vi "hReadChannels-UandP-2013.vi"(0 "FPGA VI Reference In":refnum<k20>, 1 "SavGol side points":i32=10, 3 "Use Voltage or Power for AO?":bool, 4 "order polynomial":i32=2, 5 "Nsamples":u32=10000, 6 "error in":errorcluster, 8 "output cluster":T3, 10 "variables cluster":T2) -> (2 "Fehler":bool, 13 "AdjustedArray":sgl[][](array[numeric]), 18 "single channel voltage array":dbl[](array[numeric]), 19 "real time P_rad array":dbl[](array[numeric]), 20 "FPGA VI Reference Out":refnum<k20>, 22 "PowerArray":sgl[][](array[numeric]), 25 "RawArray":sgl[][](array[numeric]), 26 "error out":errorcluster)   [LabVIEW 2014]
doc: "startet das einlesen und führt dies bis n Samples aus\nHier mit FIFO und IRQ."
uses:
  <vilib>/Utility/error.llb/Error Cluster From Error Code.vi
  <vilib>/rvi/errors/niLvFpgaAdjustHostInterfaceError.vi
  <vilib>/RVI Host/nirviSupport.llb/nirviErrorClusterFromErrorCode.vi
  <vilib>/rvi/interface/nirviReadWriteControl/nirviReadWriteControl.xnode
  FPGA Bitfiles/W7XBolo2017_FPGATarget_fmain2014_DACRangeVoltage.lvbitx
  f_main_2014.vi
  <vilib>/rvi/interface/nirviMethod/nirviMethod.xnode
  NiFpgaLv.dll
  <vilib>/rvi/interface/nirviMethod/StockFPGA_InlinedMethodWaitForMultipleIRQ.vi
  <vilib>/FPGAPlugInAG/PCI-7813R/niLvFpga_WaitOnIrq_PCI-7813R.vi
  <vilib>/FPGAPlugInAG/PCI-7813R/niLvFpga_AcknowledgeIrq_PCI-7813R.vi
  <vilib>/FPGAPlugInAG/PCI-7813R/niLvFpga_ReadFifo_PCI-7813R.vi
  <vilib>/rvi/errors/niLvFpgaMergeErrorWithErrorCode.vi
panel:
  out "channel number":i64
  in  "Tab Control":T1(tab)
  out "16bit integer voltage sample":i16[](array[numeric])
  out "RTPRad voltage factor":dbl
  out "Timed Out":bool
  out "STOP?":bool
  out "Elements Remaining":u32
  out "single channel voltage":sgl
  out "single channel voltage * factor":dbl
  out "empty sample array":dbl[](array[numeric])
  out "Nsamples array":i64[](array[numeric])
  out "dU/dt":sgl[](array[numeric])
  out "sample":i32
  out "new level of override":i32
  out "sate":string
  out "last U sample":sgl[](array[numeric])
  out "current P_rad [MW]":dbl
  out "rt prad average array":dbl[][](array[numeric])
  out "elec. channel selected":i64
  out "element of channel\nand sample":sgl
  out "column":i32
  out "channel index":i32
  out "av/f_OT*volume/k_bolo/V_cam":dbl
  out "average":dbl
  out "sum":dbl
  out "av/f_OT*volume":dbl
  out "average/f_OT":sgl
  out "av/f_OT*volume/k_bolo":dbl
  in  "magic number":dbl=1.0
  out "current power":sgl[](array[numeric])
  out "prad av array":dbl[](array[numeric])
  in  "No. Of Samples to average":i32=10
  out "index status":bool
  out "RawScal":dbl[](array[numeric])
  out "Scale(mV)":sgl[](array[numeric])
  out "SumScal":dbl[](array[numeric])
  out "Tau/dt":dbl[](array[numeric])
  out "F_ch":dbl[](array[numeric])
  out "tau_fact":dbl[](array[numeric])
  out "kbolott_and_volume":dbl[][](array[numeric])
  out "samples to exclude":u32
  out "single channel number":i64
  out "channelNumber":i32
  out "channelSelection":i64[][](array[numeric])
  out "tau_M":dbl[](array[numeric])
  out "Offsets":dbl[](array[numeric])
  out "SampleTime":sgl
  out "voltage factor":dbl
  out "Scale(mV) transf.":sgl[](array[numeric])
  out "V_cam":dbl
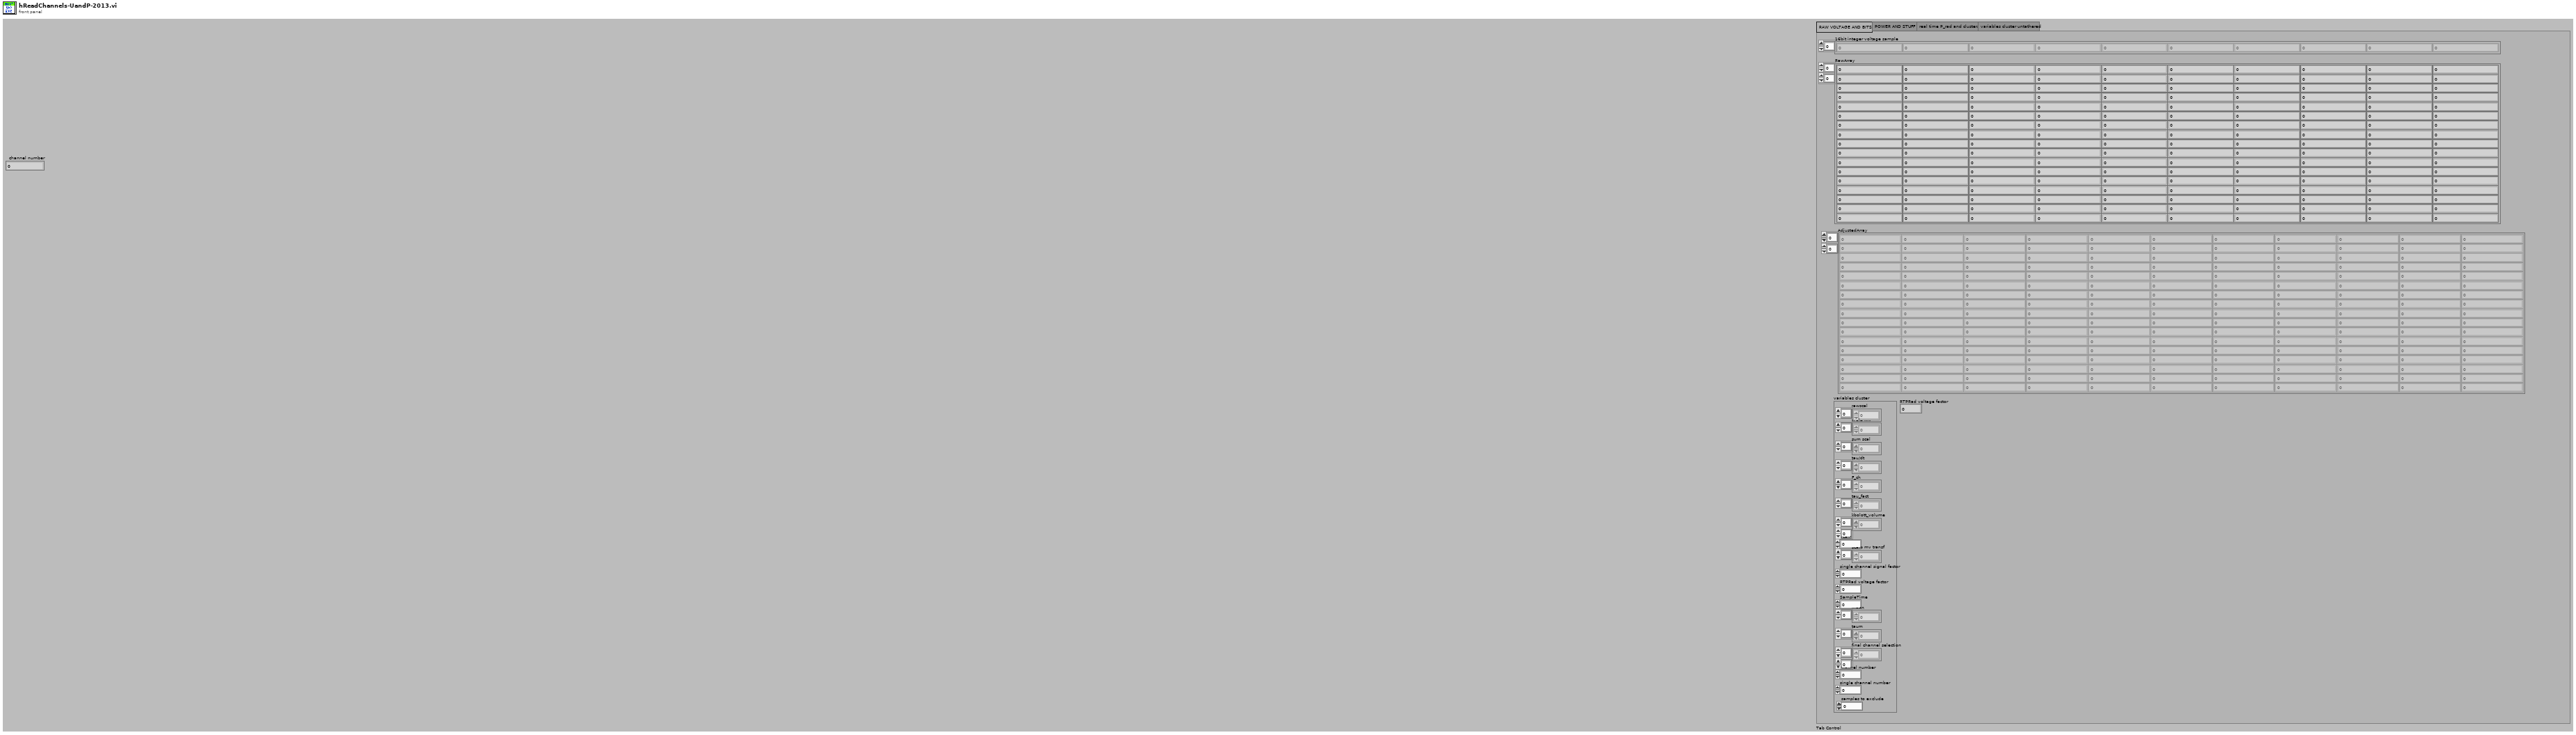
[diagram p1: front panel]
types:
  T1 = enum32{"RAW VOLTAGE AND BITS", "POWER AND STUFF", "real time P_rad and clusters", "variables cluster untathered"}
  T2 = cluster{"rawscal":dbl[], "scale mv":sgl[], "sum scal":dbl[], "tau/dt":dbl[], "F_ch":dbl[], "tau_fact":dbl[], "kbolott_volume":dbl[][], "Vcam":dbl, "scale mv transf":sgl[], "single channel signal factor":dbl, "RTPRad voltage factor":dbl, "SampleTime":sgl, "mean":dbl[], "taum":dbl[], "final channel selection":i64[][], "channel number":i32, "single channel number":i64, "samples to exclude":u32}
  T3 = cluster{"real time P_rad":refnum<vi>, "real time P_rad array":refnum<vi>, "single channel voltage":refnum<vi>, "single channel voltage array":refnum<vi>}
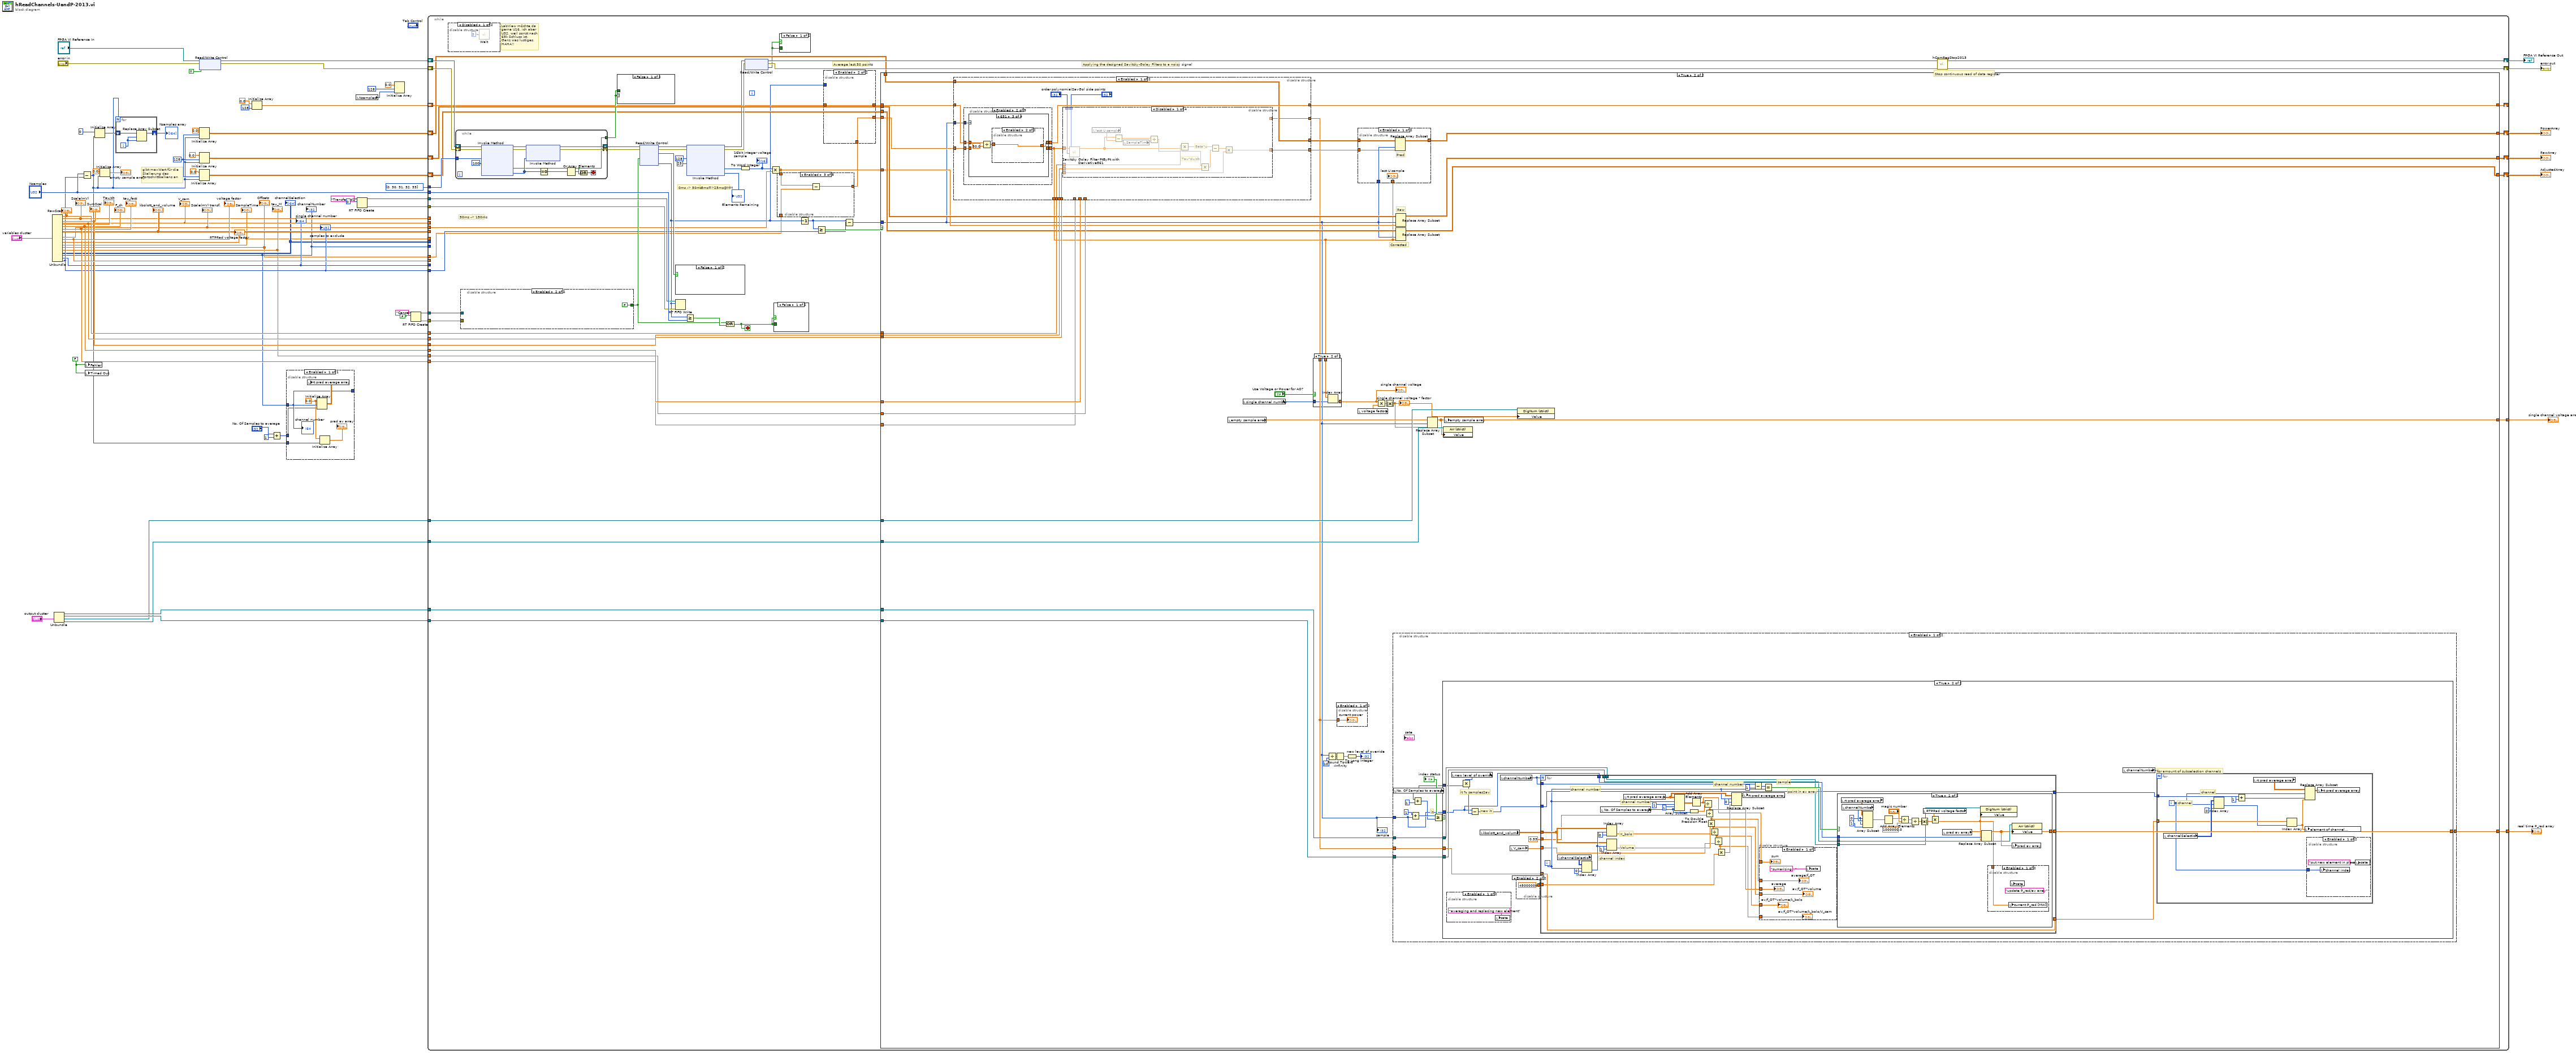
[diagram p0: block diagram]
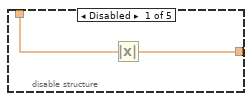
[diagram p2: hidden frame]
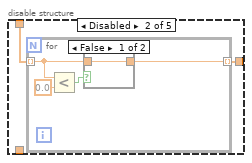
[diagram p3: hidden frame]
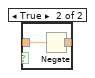
[diagram p4: hidden frame]
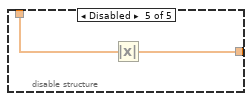
[diagram p6: hidden frame]
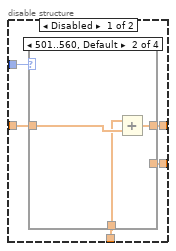
[diagram p7: hidden frame]
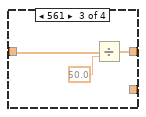
[diagram p9: hidden frame]
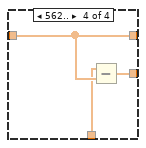
[diagram p10: hidden frame]
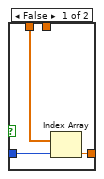
[diagram p12: hidden frame]
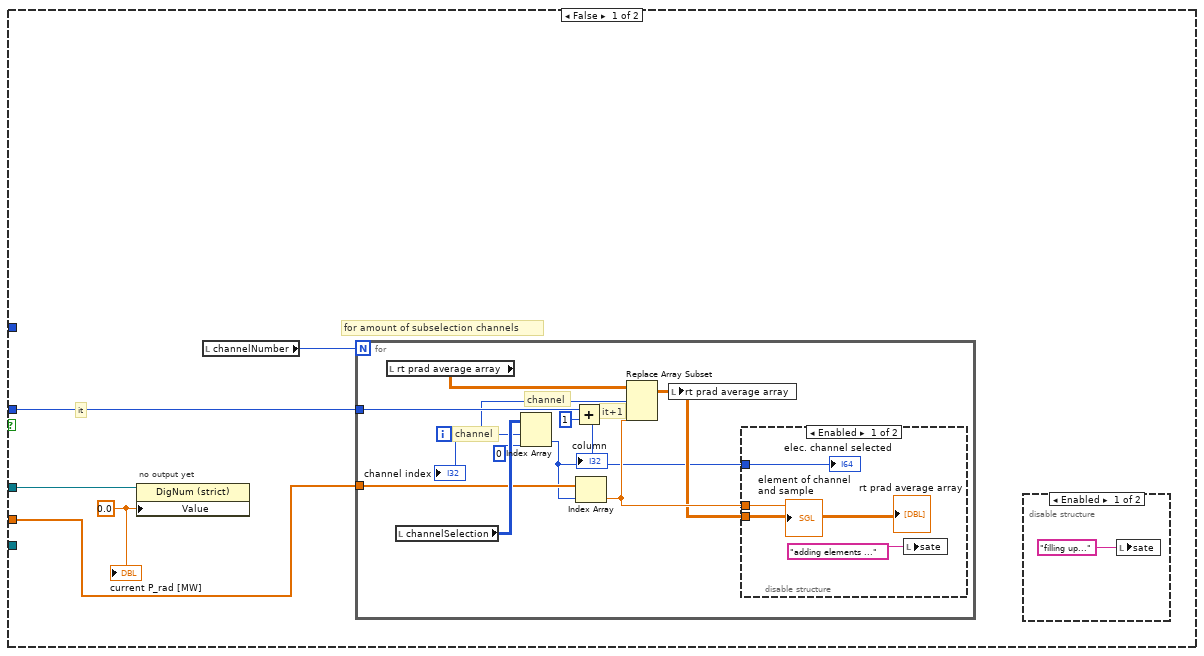
[diagram p14: hidden frame]
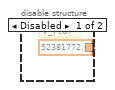
[diagram p17: hidden frame]
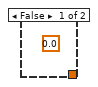
[diagram p20: hidden frame]
diagram:
  w40 = FALSE
  w14 = 128 ("dimension size")
  # "Stop continuous read of data register"
  # "gibt maxWert für die Skalierung des Fortschrittbalkens an"
  n1 = Unbundle("variables cluster") -> ("rawscal"=w31:dbl[], "scale mv"=w26:sgl[], "sum scal"=w32:dbl[], "tau/dt"=w30:dbl[], "F_ch"=w29:dbl[], "tau_fact"=w28:dbl[], "kbolott_volume"=w27:dbl[][], "Vcam"=w24:dbl, "scale mv transf"=w25:sgl[], "single channel signal factor"=w33:dbl, "RTPRad voltage factor"=→"RTPRad voltage factor":dbl, "SampleTime"=w3:sgl, "mean"=w4:dbl[], "taum"=w5:dbl[], "final channel selection"=w6:i64[][], "channel number"=w7:i32, "single channel number"=w8:i64, "samples to exclude"=w9:u32)
  "RawScal" <- w31
  "Scale(mV)" <- w26
  "SumScal" <- w32
  "Tau/dt" <- w30
  "F_ch" <- w29
  "tau_fact" <- w28
  "kbolott_and_volume" <- w27
  "V_cam" <- w24
  "Scale(mV) transf." <- w25
  "voltage factor" <- w33
  "SampleTime" <- w3
  "Offsets" <- w4
  "tau_M" <- w5
  "channelSelection" <- w6
  "channelNumber" <- w7
  "single channel number" <- w8
  "samples to exclude" <- w9
  n2 = Unbundle("output cluster") -> ("real time P_rad"=w35:refnum<vi>, "real time P_rad array"=w34:refnum<vi>, "single channel voltage"=w19:refnum<vi>, "single channel voltage array"=w18:refnum<vi>)
  n3 = Subtract(x="Nsamples", y=w9) -> (x-y=w13:u32)
  n4 = local write "Fehler"(w40) -> ()
  n5 = local write "Timed Out"(w40) -> ()
  n6 = Initialize Array(i64 0 ("element"), w13) -> (w42:i64[])
  n7 = Initialize Array(0.0 ("element"), w13) -> (→"empty sample array":dbl[])
  n8 = for {
    N: w13 -> [_]
    shift-right: [w72] -> w41
    shift-left: w42 -> [w74]
    i -> [w73]
    n9 = Replace Array Subset(array=w74, new element=w73, index=w73) -> (w72:i64[])
  }
  "Nsamples array" <- w41
  n10 = Initialize Array(sgl 0.0 ("element"), w14, w13) -> (w12:sgl[][])
  n11 = xnode "Read/Write Control"("FPGA VI Reference In"="FPGA VI Reference In", "error in"="error in", "ADCRead"=TRUE) -> ("FPGA VI Reference Out"=w53:refnum<k20>, "error out"=w52:errorcluster)
  n12 = Initialize Array(sgl 0.0 ("i"), w14, w13) -> (w62:sgl[][])
  n13 = Initialize Array(sgl 0.0, w14, w13) -> (w71:sgl[][])
  n14 = Initialize Array(sgl 0.0 ("element"), 128 ("dimension size")) -> (w48:sgl[])
  n15 = Add(x="No. Of Samples to average", y=1) -> (x+y=w21:i32)
  n16 = disable-structure shown="Enabled" {
    disable-tunnel: w7 -> [w79]
    disable-tunnel: [w79] -> _
    disable-tunnel: w21 -> [w75]
    disable-tunnel: w13 -> [w76]
    frame Enabled {
      w78 = 0.0 ("element")
      n17 = Initialize Array(w78, w79, w75) -> (w80:dbl[][])
      n18 = local write "rt prad average array"(w80) -> ()
      n19 = Initialize Array(w78, w76) -> (→"prad av array":dbl[])
      "channel number" <- w79
    }
  }
  n20 = local read "Nsamples"() -> (w37:u32)
  n21 = RT FIFO Create(0:"Transferred1" ("name (unnamed)"), 1:u32 0) -> (8:w68:refnum<k33>, 11:w67:errorcluster)  [unwired: 2 in, 5 out]
  n22 = Initialize Array(sgl 0.0 ("element"), 128 ("dimension size"), w37) -> ()  [unwired: 1 out]
  n23 = RT FIFO Create(0:"Cancel" ("name (unnamed)"), 1:FALSE) -> (8:w65:refnum<k33>, 11:w64:errorcluster)  [unwired: 2 in, 5 out]
  n24 = while {
    tunnel: "Nsamples" -> [w133]
    shift-right: [w101] -> w10
    shift-left: w71 -> [w122]
    shift-right: [w134] -> w61
    shift-left: w53 -> [w137]
    shift-right: [w135] -> w60
    shift-left: w52 -> [w136]
    tunnel: w68 -> [w132]
    tunnel: w67 -> [w131]
    tunnel: w65 -> [w129]
    tunnel: w64 -> [w128]
    shift-right: [w126] -> w56
    shift-left: w62 -> [w127]
    tunnel: w25 -> [w121]
    tunnel: w30 -> [w118]
    tunnel: w32 -> [w120]
    tunnel: w31 -> [w119]
    shift-right: [w111] -> _
    shift-left: w48 -> [w87]
    tunnel: i32[] [0, 30, 31, 32, 33] -> [w106]
    tunnel: w18 -> [w103]
    tunnel: w19 -> [w102]
    tunnel: w8 -> [_]
    tunnel: w33 -> [_]
    tunnel: w4 -> [w81]
    tunnel: w9 -> [w82]
    tunnel: w35 -> [w98]
    tunnel: w34 -> [w93]
    tunnel: w29 -> [w97]
    tunnel: w28 -> [w96]
    tunnel: w26 -> [_]
    tunnel: w27 -> [_]
    tunnel: w3 -> [_]
    tunnel: w5 -> [w95]
    tunnel: w6 -> [_]
    tunnel: w7 -> [_]
    tunnel: w24 -> [_]
    tunnel: [w92] -> w17
    tunnel: [w91] -> w16
    shift-right: [w89] -> w11
    shift-left: w12 -> [w90]
    stop <- w107 stop-if-true
    # "Average last 50 points"
    # "Applying the designed Savitzky-Golay Filters to a noisy signal"
    # "LabView möchte da gerne U16, ich aber U32, weil sonst nach 65k Schluss ist. \nGanz was lustiges, HAHA!!"
    # "5ms=>25ms@MM"
    # "0ms -> 50ms"
    # "50ms -> 150ms"
    n25 = disable-structure shown="Disabled" {
      frame Disabled {
        n26 = call "Wait"("Count(uSec)"=u32 5) -> ()  [unwired: 1 out]
      }
      frame Enabled {
      }
    }
    n27 = while {
      tunnel: [w513] -> w110
      shift-right: [w515] -> w104
      shift-left: w137 -> [w522]
      shift-right: [w514] -> w105
      shift-left: w136 -> [w521]
      tunnel: w106 -> [w519]
      stop <- w512 stop-if-true
      n28 = xnode "Invoke Method"("FPGA VI Reference In"=w522, "error in"=w521, "IRQ Number(s)"=w519, "Timeout (ms)"=100) -> ("FPGA VI Reference Out"=w516:refnum<k20>, "error out"=w517:errorcluster, "Timed Out"=w513:bool, "IRQ(s) Asserted"=w518:i32[])
      n29 = xnode "Invoke Method"("FPGA VI Reference In"=w516, "error in"=w517, "IRQ Number(s)"=w518) -> ("FPGA VI Reference Out"=w515:refnum<k20>, "error out"=w514:errorcluster)
      n30 = Equal To 0?(x=w518) -> (x = 0?=w511:bool[])
      n31 = Or Array Elements(Boolean array=w511) -> (logical OR=w510:bool)
      n32 = Or(x=w510, y=w513) -> (x .or. y?=w512:bool)
    }
    n33 = disable-structure shown="Enabled" {
      disable-tunnel: [w528 FALSE] -> w130
      disable-tunnel: w129 -> [w527 _]
      disable-tunnel: w128 -> [w526 _]
      frame Disabled {
        # "Da es passieren kann, dass der letzte IRQ verschluckt wird, sichert dies der Timeoutwert von 50ms ab."
        n34 = RT FIFO Read(0:w527, 1:FALSE ("element"), 3:w526) -> (9:w528:bool)  [unwired: 5 out]
      }
      frame Enabled {
      }
    }
    n35 = case shown="False" w110 {
      tunnel: w110 -> [_ w530]
      frame False {
      }
      frame True {
        "Timed Out" <- w530
      }
    }
    n36 = xnode "Read/Write Control"("FPGA VI Reference In"=w104, "error in"=w105, "cancel"=w130) -> ("FPGA VI Reference Out"=w124:refnum<k20>, "error out"=w123:errorcluster, "Timeout"=w125:bool, "ScanID"=w88:u32)
    n37 = case shown="False" w125 {
      selector: w125 -> [_ w532]
      frame False {
      }
      frame True {
        n38 = local write "Fehler"(w532) -> ()
      }
    }
    n39 = RT FIFO Write(0:w132, 1:w88, 3:w131) -> ()  [unwired: 1 in, 5 out]
    n40 = Greater Or Equal?(x=w88, y=w133) -> (x >= y?=w138:bool)
    n41 = xnode ("Invoke Method")("FPGA VI Reference In"=w124, "error in"=w123, "Number of Elements"=u32 128, "Timeout (ms)"=25 ("Timeout")) -> ("FPGA VI Reference Out"=w113:refnum<k20>, "error out"=w112:errorcluster, "Data"=w115:u32[], "Elements Remaining"=→"Elements Remaining":u32)
    n42 = Compound Arithmetic op=OR(w130, w138) -> (w107:bool)
    n43 = To Word Integer(number=w115) -> (16bit integer=w114:i16[])
    "16bit integer voltage sample" <- w114
    n44 = xnode "Read/Write Control"("FPGA VI Reference In"=w113, "error in"=w112) -> ("FPGA VI Reference Out"=w134:refnum<k20>, "error out"=w135:errorcluster, "Fifo-Fehler"=w108:bool)
    n45 = Multiply(x=w114, y=w121) -> (x*y=w85:sgl[])
    n46 = case shown="False" w107 {
      tunnel: w107 -> [_ w523]
      frame False {
      }
      frame True {
        "STOP?" <- w523
      }
    }
    n47 = disable-structure shown="Enabled" {
      disable-tunnel: [w140 w141 w152 w153 w155] -> w84
      disable-tunnel: w85 -> [w139 w142 w151 w153 w154]
      disable-tunnel: w81 -> [_ _ w150 _ _]
      frame Disabled {
        n48 = Absolute Value(x=w139) -> (abs(x)=w140:sgl[])
      }
      frame Disabled {
        n49 = for {
          tunnel: w142 -> [w144] mode=indexing
          tunnel: [w143] -> w141 mode=indexing
          n50 = Less?(x=w144, y=sgl 0.0) -> (x < y?=w145:bool)
          n51 = case shown="False" w145 {
            tunnel: w144 -> [w147 w149]
            tunnel: [w147 w148] -> w143
            frame False {
            }
            frame True {
              n52 = Negate(x=w149) -> (-x=w148:sgl)
            }
          }
        }
      }
      frame Enabled {
        n53 = Subtract(x=w151, y=w150) -> (x-y=w152:dbl[])
      }
      frame Disabled {
      }
      frame Disabled {
        n54 = Absolute Value(x=w154) -> (abs(x)=w155:sgl[])
      }
    }
    n55 = case shown="False" w108 {
      tunnel: w108 -> [_ w524]
      frame False {
      }
      frame True {
        "Fehler" <- w524
      }
    }
    n56 = Decrement(x=w88) -> (x-1=w99:u32)
    n57 = Greater Or Equal?(x=w99, y=w82) -> (x >= y?=w100:bool)
    n58 = disable-structure shown="Enabled" {
      disable-tunnel: [w160 w172] -> w86
      disable-tunnel: w87 -> [w159 w172]
      disable-tunnel: w88 -> [w158 _]
      disable-tunnel: [w157 w171] -> w83
      disable-tunnel: w84 -> [w156 w171]
      frame Disabled {
        n59 = case shown="501..560, Default" w158 {
          tunnel: w156 -> [_ w162 _ w168]
          tunnel: [w161 w164 w165 w169] -> w160
          tunnel: w159 -> [w161 w163 w167 w169]
          tunnel: [_ _ _ w170] -> w157
          frame 0..500 {
          }
          frame 501..560, Default {
            n60 = Add(x=w162, y=w163) -> (x+y=w164:dbl[])
          }
          frame 561 {
            n61 = Divide(x=w167, y=sgl 50.0) -> (x/y=w165:dbl[])
          }
          frame 562.. {
            n62 = Subtract(x=w168, y=w169) -> (x-y=w170:dbl[])
          }
        }
      }
      frame Enabled {
      }
    }
    n63 = Subtract(x=w99, y=w82) -> (x-y=w94:u32)
    n64 = case shown="True" w100 {
      tunnel: w127 -> [w175 w214]
      tunnel: [w175 w207] -> w126
      tunnel: w122 -> [w174 w205]
      tunnel: w120 -> [_ w213]
      tunnel: w119 -> [_ w212]
      tunnel: w118 -> [_ w211]
      tunnel: [w176 w210] -> w111
      tunnel: w86 -> [w176 w184]
      tunnel: w85 -> [_ w183]
      tunnel: w103 -> [_ w209]
      tunnel: w102 -> [_ w208]
      tunnel: [w174 w204] -> w101
      tunnel: w94 -> [_ w181]
      tunnel: w98 -> [_ w200]
      tunnel: w93 -> [_ w199]
      tunnel: w97 -> [_ w203]
      tunnel: w96 -> [_ w201]
      tunnel: w95 -> [_ w202]
      tunnel: [_ w189] -> w92
      tunnel: [_ w188] -> w91
      tunnel: w90 -> [w173 w186]
      tunnel: [w173 w185] -> w89
      tunnel: w83 -> [_ w182]
      frame False {
      }
      frame True {
        # "Corrected"
        # "Raw"
        n65 = disable-structure shown="Enabled" {
          disable-tunnel: w214 -> [w362 w477]
          disable-tunnel: w213 -> [w369 _]
          disable-tunnel: w212 -> [w368 _]
          disable-tunnel: w211 -> [w367 _]
          disable-tunnel: [w366 w473] -> w210
          disable-tunnel: w184 -> [w365 w475]
          disable-tunnel: w182 -> [w359 w474]
          disable-tunnel: w181 -> [w364 w476]
          disable-tunnel: w202 -> [_ w483]
          disable-tunnel: w203 -> [_ w482]
          disable-tunnel: w201 -> [_ w481]
          disable-tunnel: [w363 w479] -> w178
          disable-tunnel: [w362 w477] -> w206
          disable-tunnel: [w358 _] -> w179
          disable-tunnel: [w357 _] -> w177
          frame Enabled {
            n66 = disable-structure shown="Enabled" {
              disable-tunnel: [w374 w400 w422] -> w366
              disable-tunnel: w365 -> [w373 w399 w422]
              disable-tunnel: w364 -> [w372 w398 _]
              disable-tunnel: [w371 w397 w423] -> w358
              disable-tunnel: w359 -> [w370 w396 w423]
              frame Disabled {
                n67 = case shown="11..60, Default" w372 {
                  tunnel: w370 -> [_ w376 _ w392]
                  tunnel: [w375 w378 w380 w391] -> w374
                  tunnel: w373 -> [w375 w377 w382 w391]
                  tunnel: [_ _ _ w390] -> w371
                  frame 0..10 {
                  }
                  frame 11..60, Default {
                    # "Average last 50 points"
                    n68 = Add(x=w376, y=w377) -> (x+y=w378:dbl[])
                  }
                  frame 61 {
                    n69 = Divide(x=w382, y=sgl 50.0) -> (x/y=w379:dbl[])
                    n70 = disable-structure shown="Enabled" {
                      disable-tunnel: [w383 w388] -> w380
                      disable-tunnel: w379 -> [w387 w388]
                      frame Disabled {
                        n71 = Initialize Array(2e-06 ("element"), 128 ("dimension size")) -> (w384:dbl[])
                        n72 = Subtract(x=w387, y=w384) -> (x-y=w383:dbl[])
                      }
                      frame Enabled {
                      }
                    }
                  }
                  frame 62.. {
                    n73 = Subtract(x=w392, y=w391) -> (x-y=w389:dbl[])
                    n74 = disable-structure shown="Enabled" {
                      disable-tunnel: [w394 w395] -> w390
                      disable-tunnel: w389 -> [w393 w395]
                      frame Disabled {
                        n75 = Absolute Value(x=w393) -> (abs(x)=w394:dbl[])
                      }
                      frame Enabled {
                      }
                    }
                  }
                }
              }
              frame Enabled {
                n76 = case shown="651" w398 {
                  tunnel: w396 -> [_ w402 _ w418]
                  tunnel: [w401 w404 w406 w417] -> w400
                  tunnel: w399 -> [w401 w403 w408 w417]
                  tunnel: [_ _ _ w416] -> w397
                  frame 0..600 {
                  }
                  frame 601..650, Default {
                    # "Average last 50 points"
                    n77 = Add(x=w402, y=w403) -> (x+y=w404:dbl[])
                  }
                  frame 651 {
                    n78 = Divide(x=w408, y=sgl 50.0) -> (x/y=w405:dbl[])
                    n79 = disable-structure shown="Enabled" {
                      disable-tunnel: [w409 w414] -> w406
                      disable-tunnel: w405 -> [w413 w414]
                      frame Disabled {
                        n80 = Initialize Array(2e-06 ("element"), 128 ("dimension size")) -> (w410:dbl[])
                        n81 = Subtract(x=w413, y=w410) -> (x-y=w409:dbl[])
                      }
                      frame Enabled {
                      }
                    }
                  }
                  frame 652.. {
                    n82 = Subtract(x=w418, y=w417) -> (x-y=w415:dbl[])
                    n83 = disable-structure shown="Enabled" {
                      disable-tunnel: [w420 w421] -> w416
                      disable-tunnel: w415 -> [w419 w421]
                      frame Disabled {
                        n84 = Absolute Value(x=w419) -> (abs(x)=w420:dbl[])
                      }
                      frame Enabled {
                      }
                    }
                  }
                }
              }
              frame Disabled {
              }
            }
            n85 = disable-structure shown="Disabled" {
              disable-tunnel: w369 -> [w438 w450 w456 _]
              disable-tunnel: w368 -> [w437 w449 w451 _]
              disable-tunnel: w367 -> [w436 w448 w455 _]
              disable-tunnel: [w435 w439 w470 w471] -> w363
              disable-tunnel: w358 -> [w434 w447 w469 w471]
              disable-tunnel: "SavGol side points" -> [w428 w442 w463 _]
              disable-tunnel: "order polynomial" -> [w429 w443 w464 _]
              disable-tunnel: [_ w439 w453 w471] -> w357
              frame Disabled {
                # "Beta*u"
                # "Tau*du/dt"
                n86 = call "Savitzky Golay Filter PtByPt with Derivative861.vi"("order polynomial"=w429, "side points"=w428, "x"=w434) -> ("Filtered x"=w424:dbl[])  [unwired: 1 in, 7 out]
                n87 = local read "last U sample"() -> (w426:sgl[])
                n88 = Subtract(x=w424, y=w426) -> (x-y=w427:dbl[])
                n89 = local read "SampleTime"() -> (w425:sgl)
                n90 = Divide(x=w427, y=w425) -> (x/y=w431:dbl[])
                n91 = Multiply(x=w437, y=w424) -> (x*y=w433:dbl[])
                n92 = Multiply(x=w431, y=w436) -> (x*y=w430:dbl[])
                n93 = Subtract(x=w433, y=w430) -> (x-y=w432:dbl[])
                n94 = Multiply(x=w432, y=w438) -> (x*y=w435:dbl[])
              }
              frame Enabled {
                # "Beta*u"
                # "Tau*du/dt"
                n95 = call "Savitzky Golay Filter PtByPt with Derivative861.vi"("order polynomial"=w443, "side points"=w442, "x"=w447) -> ("Filtered Derivative"=w440:dbl[], "Filtered x"=w441:dbl[])  [unwired: 1 in, 6 out]
                n96 = Multiply(x=w449, y=w441) -> (x*y=w446:dbl[])
                n97 = Multiply(x=w440, y=w448) -> (x*y=w444:dbl[])
                n98 = Subtract(x=w446, y=w444) -> (x-y=w445:dbl[])
                n99 = Multiply(x=w445, y=w450) -> (x*y=w439:dbl[])
              }
              frame Disabled {
                # "Beta*u"
                # "Tau*du/dt"
                n100 = call "Savitzky Golay Filter PtByPt with Derivative861.vi"("order polynomial"=w464, "side points"=w463, "x"=w469) -> ("Filtered Derivative"=w454:dbl[], "Filtered x"=w452:dbl[])  [unwired: 1 in, 6 out]
                n101 = local read "last U sample"() -> (w461:sgl[])
                n102 = Subtract(x=w452, y=w461) -> (x-y=w462:dbl[])
                n103 = local read "SampleTime"() -> (w460:sgl)
                n104 = Divide(x=w462, y=w460) -> (x/y=w466:dbl[])
                n105 = Multiply(x=w451, y=w452) -> (x*y=w459:dbl[])
                n106 = Multiply(x=w451, y=w452) -> (x*y=w468:dbl[])
                n107 = Multiply(x=w454, y=w455) -> (x*y=w457:dbl[])
                n108 = Multiply(x=w466, y=w455) -> (x*y=w465:dbl[])
                n109 = Subtract(x=w459, y=w457) -> (x-y=w458:dbl[])
                n110 = Subtract(x=w468, y=w465) -> (x-y=w467:dbl[])
                n111 = Multiply(x=w458, y=w456) -> (x*y=w453:dbl[])
                n112 = Multiply(x=w467, y=w456) -> (x*y=w470:dbl[])
              }
              frame Disabled {
              }
            }
          }
          frame Disabled {
            # "beta=[1-(omega*R_ch)^2+(omega*r_C)^2]/\n         {1+[omega*{R_ch+r_C}]^2}"
            # "tau_fact[((1-U_eff^2*beta)/4)/kappa_ch]/{R_ch+r_C}^2"
            # "U_eff=(U_0*R_Ch)/(R_ch+2*r_C)"
            # "omega=2*Pi*f_bridge*C_Cab"
            # "=2/U_eff * (R_ch+r_C)*kappa_ch\n  * sqrt(1+[omega+(R_ch+r_C)]^2)\n  * {tau_ch*dU/dt+tau_fact*U_ch}"
            # "P_ch=F_Ch*(tau_ch*dU/dt+tau_fact*U_ch)"
            # "tau_channels"
            # "F_ch"
            # "tau_fact"
            # "U_raw"
            # "dU/dt"
            n113 = case shown="62.." w476 {
              tunnel: w474 -> [_ w491 _ w497]
              tunnel: [w489 w492 w494 w498] -> w473
              tunnel: w475 -> [w489 w490 w495 w498]
              tunnel: [w489 _ _ w496] -> w472
              frame 0..10 {
              }
              frame 11..60, Default {
                # "Average last 50 points"
                n114 = Add(x=w491, y=w490) -> (x+y=w492:dbl[])
              }
              frame 61 {
                n115 = Divide(x=w495, y=sgl 50.0) -> (x/y=w494:dbl[])
              }
              frame 62.. {
                n116 = Subtract(x=w497, y=w498) -> (x-y=w496:dbl[])
              }
            }
            n117 = local read "last U sample"() -> (w478:sgl[])
            n118 = local read "SampleTime"() -> (w480:sgl)
            n119 = disable-structure shown="Enabled" {
              disable-tunnel: w472 -> [w504 w505]
              disable-tunnel: [w503 w506] -> w485
              disable-tunnel: [w500 w505] -> w484
              disable-tunnel: w478 -> [_ w509]
              disable-tunnel: w480 -> [_ w507]
              frame Enabled {
                n120 = call "Savitzky Golay Filter PtByPt with Derivative861.vi"("order polynomial"=2, "side points"=11, "x"=w504) -> ("Filtered Derivative"=w503:dbl[], "Filtered x"=w500:dbl[])  [unwired: 1 in, 6 out]
              }
              frame Disabled {
                # "differentiation"
                n121 = Subtract(x=w505, y=w509) -> (x-y=w508:dbl[])
                n122 = Divide(x=w508, y=w507) -> (x/y=w506:dbl[])
              }
            }
            n123 = disable-structure shown="Enabled" {
              disable-tunnel: w485 -> [w499 _]
              frame Enabled {
                "dU/dt" <- w499
              }
              frame Disabled {
              }
            }
            n124 = Multiply(x=w484, y=w481) -> (x*y=w488:dbl[])
            n125 = Multiply(x=w485, y=w483) -> (x*y=w486:dbl[])
            n126 = Add(x=w488, y=w486) -> (x+y=w487:dbl[])
            n127 = Multiply(x=w487, y=w482) -> (x*y=w479:dbl[])
          }
        }
        n128 = local read "empty sample array"() -> (w196:dbl[])
        n129 = local read "single channel number"() -> (w198:i64)
        n130 = case shown="True" "Use Voltage or Power for AO?" {
          tunnel: w198 -> [w215 w220]
          tunnel: [w216 w219] -> w195
          tunnel: w179 -> [_ w218]
          tunnel: w177 -> [w217 _]
          frame False {
            n131 = Index Array(array=w217, index=w215) -> (element=w216:dbl)
          }
          frame True {
            n132 = Index Array(array=w218, index=w220) -> (element=w219:dbl)
          }
        }
        "single channel voltage" <- w195
        n133 = Divide(x=w181, y=10) -> (x/y=w191:dbl)
        n134 = Round Toward -Infinity(1:w191) -> (0:w192:dbl)
        n135 = disable-structure shown="Enabled" {
          disable-tunnel: w177 -> [w221 _]
          frame Enabled {
            "current power" <- w221
          }
          frame Disabled {
          }
        }
        n136 = To Long Integer(number=w192) -> (32bit integer=→"new level of override":i32)
        n137 = disable-structure shown="Enabled" {
          disable-tunnel: w206 -> [w355 w356]
          disable-tunnel: [w354 w356] -> w207
          disable-tunnel: w181 -> [w353 _]
          disable-tunnel: w178 -> [w352 _]
          disable-tunnel: w179 -> [w351 _]
          frame Enabled {
            # "Prad"
            n138 = Replace Array Subset(array=w355, new element=w352, index (col)=w353) -> (w354:sgl[][])  [unwired: 1 in]
            "last U sample" <- w351
          }
          frame Disabled {
          }
        }
        n139 = local read "voltage factor"() -> (w197:dbl)
        n140 = Multiply(x=w195, y=w197) -> (x*y=w194:dbl)
        n141 = Absolute Value(x=w194) -> (abs(x)=w180:dbl)
        "single channel voltage * factor" <- w180
        n142 = disable-structure shown="Enabled" {
          disable-tunnel: w181 -> [w226 _]
          disable-tunnel: w200 -> [w229 _]
          disable-tunnel: w199 -> [w228 _]
          disable-tunnel: w177 -> [w227 _]
          disable-tunnel: [w222 _] -> w189
          frame Enabled {
            # "it"
            n143 = local read "No. Of Samples to average"() -> (w223:i32)
            n144 = Add(x=1, y=w226) -> (x+y=w230:u32)
            n145 = Add(x=w223, y=i64 1) -> (x+y=w224:i64)
            n146 = Greater Or Equal?(x=w230, y=w224) -> (x >= y?=w232:bool)
            "index status" <- w232
            n147 = case shown="True" w232 {
              tunnel: w226 -> [w233 w256]
              tunnel: w229 -> [w236 w258]
              tunnel: w228 -> [_ w259]
              tunnel: w227 -> [w234 w257]
              tunnel: w223 -> [_ w255]
              tunnel: [_ w254] -> w222
              frame False {
                w235 = 0.0 ("Value")
                # "it"
                # "for amount of subselection channels"
                # "no output yet"
                n148 = property class="DigNum (strict)"(reference=w236, "Value"=w235) -> ()  [unwired: 1 in, 2 out]
                n149 = local read "channelNumber"() -> (w237:i32)
                n150 = for {
                  N: w237 -> [_]
                  tunnel: w233 -> [w245]
                  tunnel: w234 -> [w243]
                  i -> [w240]
                  # "channel"
                  # "channel"
                  # "it+1"
                  n151 = local read "rt prad average array"() -> (w244:dbl[][])
                  n152 = local read "channelSelection"() -> (w249:i64[][])
                  n153 = Index Array(array=w249, index (row)=w240, index (col)=0 ("disabled index (col)")) -> (element=w239:i64)
                  n154 = Add(x=w245, y=1) -> (x+y=w246:u32)
                  "column" <- w246
                  n155 = Index Array(array=w243, index=w239) -> (element=w242:dbl)
                  n156 = Replace Array Subset(array=w244, new element=w242, index (row)=w240, index (col)=w246) -> (w241:dbl[][])
                  n157 = local write "rt prad average array"(w241) -> ()
                  n158 = disable-structure shown="Enabled" {
                    disable-tunnel: w239 -> [w252 _]
                    disable-tunnel: w242 -> [w251 _]
                    disable-tunnel: w241 -> [w250 _]
                    frame Enabled {
                      n159 = local write "sate"("adding elements ...") -> ()
                      "element of channel\nand sample" <- w251
                      "elec. channel selected" <- w252
                      "rt prad average array" <- w250
                    }
                    frame Disabled {
                    }
                  }
                  "channel index" <- w240
                }
                n160 = disable-structure shown="Enabled" {
                  frame Enabled {
                    n161 = local write "sate"("filling up...") -> ()
                  }
                  frame Disabled {
                  }
                }
                "current P_rad [MW]" <- w235
              }
              frame True {
                # "new it"
                # "it % samples2av"
                # "for amount of subselection channels"
                n162 = disable-structure shown="Enabled" {
                  frame Enabled {
                    n163 = local write "sate"("averaging and replacing new element") -> ()
                  }
                  frame Disabled {
                  }
                }
                n164 = local read "new level of override"() -> (w269:i32)
                n165 = Multiply(x=w269, y=w255) -> (x*y=w268:i32)
                n166 = Subtract(x=w256, y=w268) -> (x-y=w266:u32)
                n167 = local read "kbolott_and_volume"() -> (w267:dbl[][])
                n168 = local read "channelNumber"() -> (w261:i32)
                n169 = local read "V_cam"() -> (w263:dbl)
                n170 = disable-structure shown="Enabled" {
                  disable-tunnel: [52381772.0 45000000.0] -> w265
                  frame Disabled {
                    # "V_Ptor"
                  }
                  frame Enabled {
                  }
                }
                n171 = for {
                  N: w261 -> [_]
                  tunnel: w267 -> [w305]
                  tunnel: [w310] -> w262
                  tunnel: w257 -> [w310]
                  tunnel: [w290] -> w260
                  tunnel: w266 -> [w290]
                  tunnel: w265 -> [w284]
                  tunnel: 0.53 -> [w288]
                  tunnel: w263 -> [w285]
                  tunnel: w261 -> [w291]
                  tunnel: w256 -> [w296]
                  tunnel: w259 -> [w295]
                  tunnel: w258 -> [w292]
                  tunnel: [w274] -> w254
                  i -> [w289]
                  # "channel number"
                  # "channel number"
                  # "point in av array"
                  # "sample"
                  # "channel number"
                  # "K_bolo"
                  # "Volume"
                  # "channel index"
                  n172 = local read "channelSelection"() -> (w309:i64[][])
                  n173 = Index Array(array=w309, index (row)=w289, index (col)=0 ("disabled index (col)")) -> (element=w306:i64)
                  n174 = local read "No. Of Samples to average"() -> (w276:i32)
                  n175 = Index Array(array=w305, index (row)=w306, index (col)=0 ("disabled index (col)")) -> (element=w286:dbl)
                  n176 = Index Array(array=w305, index (row)=w306, index (col)=1 ("disabled index (col)")) -> (element=w287:dbl)
                  n177 = local read "rt prad average array"() -> (w300:dbl[][])
                  n178 = Array Subset(array=w300, index (row)=w289, length (row)=1, index (col)=1 ("index"), length (col)=w276) -> (w301:dbl[][])
                  n179 = To Double Precision Float(number=w276) -> (double precision float=w275:dbl)
                  n180 = Add Array Elements(numeric array=w301) -> (sum=w281:dbl)
                  n181 = Divide(x=w281, y=w275) -> (x/y=w282:dbl)
                  n182 = Divide(x=w282, y=w288) -> (x/y=w280:dbl)
                  n183 = Multiply(x=w280, y=w287) -> (x*y=w279:dbl)
                  n184 = Divide(x=w279, y=w286) -> (x/y=w278:dbl)
                  n185 = Divide(x=w278, y=w285) -> (x/y=w277:dbl)
                  n186 = Multiply(x=w277, y=w284) -> (x*y=w283:dbl)
                  n187 = Replace Array Subset(array=w300, new element=w283, index (row)=w289, index (col)=0 ("disabled index (col)")) -> (w298:dbl[][])
                  n188 = local write "rt prad average array"(w298) -> ()
                  n189 = Subtract(x=w291, y=i64 1) -> (x-y=w294:i64)
                  n190 = disable-structure shown="Enabled" {
                    disable-tunnel: w282 -> [w316 _]
                    disable-tunnel: w281 -> [w315 _]
                    disable-tunnel: w280 -> [w314 _]
                    disable-tunnel: w279 -> [w313 _]
                    disable-tunnel: w278 -> [w312 _]
                    disable-tunnel: w277 -> [w311 _]
                    frame Enabled {
                      n191 = local write "sate"("sumarizing...") -> ()
                      "av/f_OT*volume/k_bolo" <- w312
                      "average/f_OT" <- w314
                      "av/f_OT*volume" <- w313
                      "sum" <- w315
                      "average" <- w316
                      "av/f_OT*volume/k_bolo/V_cam" <- w311
                    }
                    frame Disabled {
                    }
                  }
                  n192 = Equal?(x=w294, y=w289) -> (x = y?=w297:bool)
                  n193 = case shown="True" w297 {
                    tunnel: w296 -> [_ w332]
                    tunnel: w295 -> [_ w331]
                    tunnel: w292 -> [_ w330]
                    tunnel: [_ w321] -> w274
                    frame False {
                      (unwired) 0.0
                    }
                    frame True {
                      w327 = 0 ("index")
                      n194 = local read "rt prad average array"() -> (w333:dbl[][])
                      n195 = local read "channelNumber"() -> (w328:i32)
                      n196 = Array Subset(array=w333, index (row)=w327, length (row)=w328, index (col)=w327, length (col)=1 ("index")) -> (w335:dbl[][])
                      n197 = Add Array Elements(numeric array=w335) -> (sum=w325:dbl)
                      n198 = Divide(x=w325, y="magic number") -> (x/y=w326:dbl)
                      n199 = Divide(x=w326, y=1000000.0) -> (x/y=w322:dbl)
                      n200 = Absolute Value(x=w322) -> (abs(x)=w320:dbl)
                      n201 = local read "RTPRad voltage factor"() -> (w318:dbl)
                      n202 = Multiply(x=w318, y=w320) -> (x*y=w319:dbl)
                      n203 = local read "prad av array"() -> (w323:dbl[])
                      n204 = property class="DigNum (strict)"(reference=w330, "Value"=w319) -> ()  [unwired: 1 in, 2 out]
                      n205 = Replace Array Subset(array=w323, new element=w319, index=w332) -> (w321:dbl[])
                      n206 = disable-structure shown="Enabled" {
                        disable-tunnel: w319 -> [w336 _]
                        frame Enabled {
                          n207 = local write "current P_rad [MW]"(w336) -> ()
                          n208 = local write "sate"("update P_rad/av array") -> ()
                        }
                        frame Disabled {
                        }
                      }
                      n209 = property class="Arr (strict)"(reference=w331, "Value"=w321) -> ()  [unwired: 1 in, 2 out]
                      n210 = local write "prad av array"(w321) -> ()
                    }
                  }
                }
                n211 = local read "channelNumber"() -> (w270:i32)
                n212 = for {
                  N: w270 -> [_]
                  tunnel: w260 -> [w344]
                  tunnel: w262 -> [w342]
                  i -> [w340]
                  # "channel"
                  # "channel"
                  n213 = local read "channelSelection"() -> (w348:i64[][])
                  n214 = Index Array(array=w348, index (row)=w340, index (col)=0 ("disabled index (col)")) -> (element=w338:i64)
                  n215 = Add(x=w344, y=1) -> (x+y=w345:u32)
                  n216 = local read "rt prad average array"() -> (w343:dbl[][])
                  n217 = Index Array(array=w342, index=w338) -> (element=w339:dbl)
                  n218 = local write "element of channel\nand sample"(w339) -> ()
                  n219 = Replace Array Subset(array=w343, new element=w339, index (row)=w340, index (col)=w345) -> (w341:dbl[][])
                  n220 = disable-structure shown="Enabled" {
                    disable-tunnel: w340 -> [w349 _]
                    frame Enabled {
                      n221 = local write "channel index"(w349) -> ()
                      n222 = local write "sate"("put new element in place") -> ()
                    }
                    frame Disabled {
                    }
                  }
                  n223 = local write "rt prad average array"(w341) -> ()
                }
              }
            }
          }
          frame Disabled {
          }
        }
        n224 = Replace Array Subset(array=w205, new element=w183, index (col)=w181) -> (w204:sgl[][])  [unwired: 1 in]
        n225 = Replace Array Subset(array=w186, new element=w179, index (col)=w181) -> (w185:sgl[][])  [unwired: 1 in]
        n226 = Replace Array Subset(array=w196, new element=w180, index=w181) -> (w188:dbl[])
        n227 = property class="Arr (strict)"(reference=w209, "Value"=w188) -> ()  [unwired: 1 in, 2 out]
        n228 = local write "empty sample array"(w188) -> ()
        n229 = property class="DigNum (strict)"(reference=w208, "Value"=w180) -> ()  [unwired: 1 in, 2 out]
        "sample" <- w181
      }
    }
  }
  "RawArray" <- w10
  "PowerArray" <- w56
  "real time P_rad array" <- w17
  "single channel voltage array" <- w16
  "AdjustedArray" <- w11
  n230 = call "hComRegStop2013.vi"("error in"=w60, "FPGA VI Reference In"=w61) -> ("error out"=→"error out":errorcluster, "FPGA VI Reference Out"=→"FPGA VI Reference Out":refnum<k20>)  [unwired: 3 in, 1 out]
